vi "Synthesize.vi"(0 "ToneCloud in":refnum<class "Tone Cloud.lvclass">, 5 "Fs (Hz)":dbl, 7 "Npts":i32, 9 "Repetition":i32, 11 "error in (no error)":errorcluster) -> (4 "ToneCloud out":refnum<class "Tone Cloud.lvclass">, 8 "Array":dbl[](array[numeric]), 15 "error out":errorcluster)   [LabVIEW 2020, in "Tone Cloud.lvclass"]
uses:
  Tone Cloud.lvclass
  Tone Cloud.lvclass/Tone Cloud.ctl
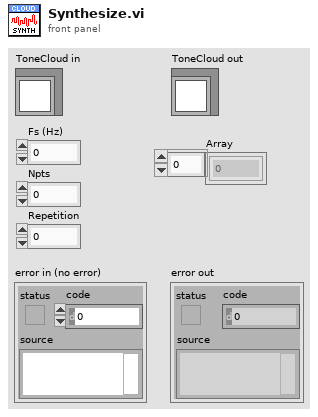
[diagram p1: front panel]
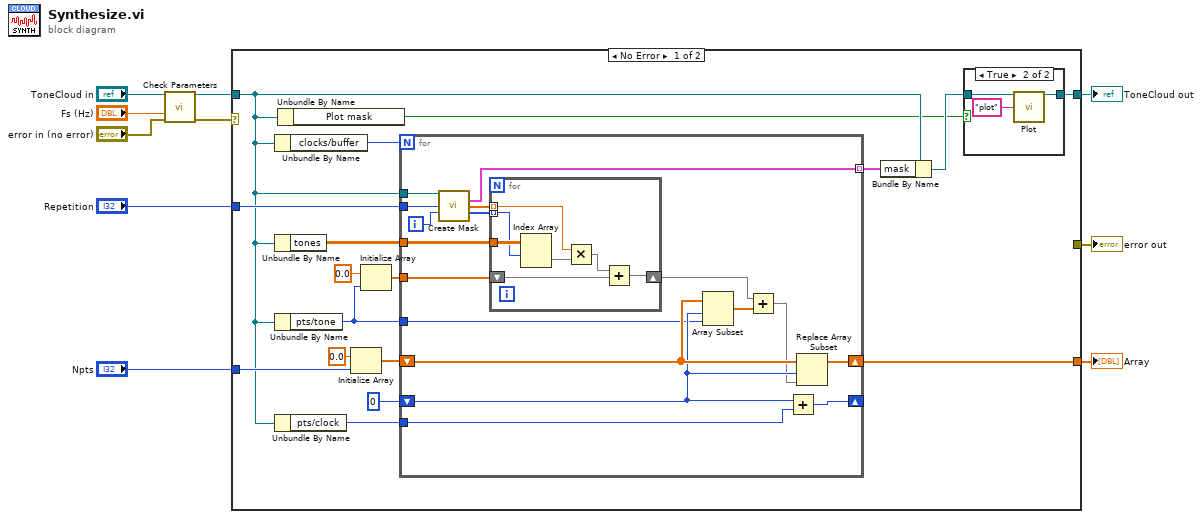
[diagram p0: block diagram]
diagram:
  n1 = call "Check Parameters.vi"("ToneCloud in"="ToneCloud in", "Fs (Hz)"="Fs (Hz)", "error in (no error)"="error in (no error)") -> ("ToneCloud out"=w4:refnum<class "Tone Cloud.lvclass">, "error out"=w1:errorcluster)  [unwired: 11 in]
  n2 = case shown="No Error" w1 {
    selector: w1 -> [_ w56]
    tunnel: [w13 w57] -> w10
    tunnel: w4 -> [w12 w57]
    tunnel: "Npts" -> [w27 _]
    tunnel: [w24 _] -> w8
    tunnel: [_ w56] -> w7
    tunnel: "Repetition" -> [w16 _]
    frame No Error {
      n3 = Unbundle By Name(w12) -> ("clocks/buffer"=w22:i32)
      n4 = Unbundle By Name(w12) -> ("tones"=w21:dbl[][])
      n5 = Unbundle By Name(w12) -> ("pts/tone"=w19:i32)
      n6 = Unbundle By Name(w12) -> ("pts/clock"=w20:i32)
      n7 = Unbundle By Name(w12) -> ("Plot mask"=w11:bool)
      n8 = Initialize Array(0.0 ("element"), w27) -> (w25:dbl[])
      n9 = Initialize Array(0.0 ("element"), w19) -> (w17:dbl[])
      n10 = for {
        N: w22 -> [_]
        shift-right: [w46] -> w24
        shift-left: w25 -> [w47]
        tunnel: w21 -> [w48]
        shift-right: [w44] -> _
        shift-left: 0 -> [w45]
        tunnel: w19 -> [w43]
        tunnel: w12 -> [w42]
        tunnel: w20 -> [w41]
        tunnel: w17 -> [w38]
        tunnel: w16 -> [w36]
        tunnel: [w32] -> w15 mode=indexing
        i -> [w35]
        n11 = call "Create Mask.vi"("ToneCloud in"=w42, "iRep"=w36, "iRow"=w35) -> ("row"=w32:cluster{"index":i32[], "level":dbl[]}, "amplitudes"=w33:dbl[], "indices"=w34:i32[])  [unwired: 8 in, 2 out]
        n12 = for {
          tunnel: w48 -> [w55]
          tunnel: w34 -> [w54] mode=indexing
          shift-right: [w53] -> w37
          shift-left: w38 -> [w52]
          tunnel: w33 -> [w49] mode=indexing
          n13 = Index Array(array=w55, index (row)=w54) -> (element=w51:dbl[])  [unwired: 1 in]
          n14 = Multiply(x=w49, y=w51) -> (x*y=w50:dbl[])
          n15 = Add(x=w50, y=w52) -> (x+y=w53:dbl[])
        }
        n16 = Array Subset(array=w47, index=w45, length=w43) -> (w40:dbl[])
        n17 = Add(x=w37, y=w40) -> (x+y=w39:dbl[])
        n18 = Add(x=w45, y=w41) -> (x+y=w44:i32)
        n19 = Replace Array Subset(array=w47, new element=w39, index=w45) -> (w46:dbl[])
      }
      n20 = Bundle By Name(cluster=w12, "mask"=w15) -> (w14:refnum<class "Tone Cloud.lvclass">)
      n21 = case shown="True" w11 {
        tunnel: w14 -> [w28 w31]
        tunnel: [w28 w30] -> w13
        frame False {
        }
        frame True {
          n22 = call "Plot.vi"("ToneCloud in"=w31, "action"="plot") -> ("ToneCloud out"=w30:refnum<class "Tone Cloud.lvclass">)  [unwired: 12 in, 1 out]
        }
      }
    }
    frame Error {
    }
  }
  "error out" <- w7
  "ToneCloud out" <- w10
  "Array" <- w8
